vi "Do.vi"(8 "error in (no error)":errorcluster, 10 "Message in":refnum<class "Interface Message.lvclass">, 11 "Execute":refnum<class "Execute.lvclass">) -> (0 "error out":errorcluster, 2 "Message out":refnum<class "Interface Message.lvclass">, 3 "Execute":refnum<class "Execute.lvclass">)   [LabVIEW 2018, in "QMH_Class.lvlib" / "TestManager.lvlib" / "Interface Message.lvclass"]
uses:
  Interface Message.lvclass
  Execute_class/Execute.lvclass
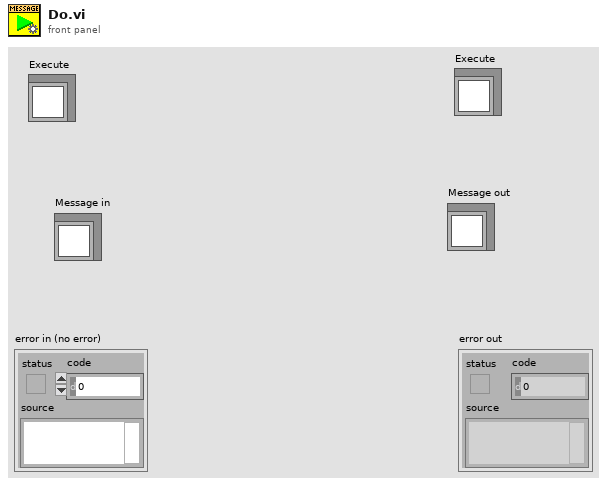
[diagram p1: front panel]
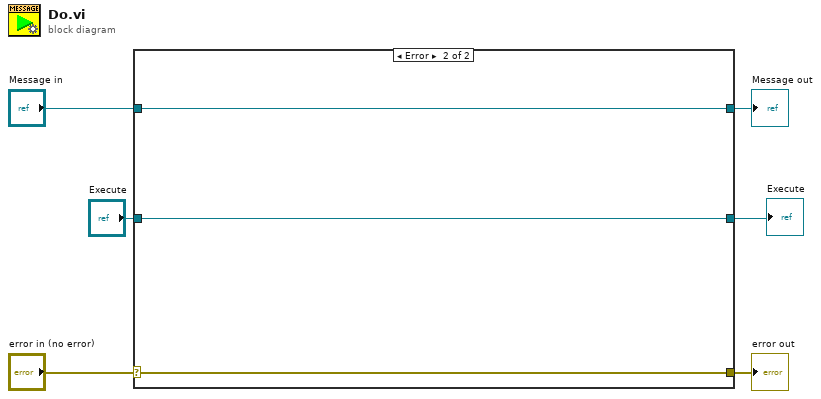
[diagram p0: block diagram]
diagram:
  n1 = case shown="Error" "error in (no error)" {
    selector: "error in (no error)" -> [w8 w12]
    tunnel: [w8 w12] -> w5
    tunnel: [w9 w11] -> w3
    tunnel: "Message in" -> [w9 w11]
    tunnel: "Execute" -> [w7 w10]
    tunnel: [w7 w10] -> w1
    frame No Error {
      # "Wire the error cluster across even in the \"No Error\"\ncase so that warnings get propagated."
    }
    frame Error {
    }
  }
  "error out" <- w5
  "Message out" <- w3
  "Execute" <- w1
